vi "Actor Core.vi"(8 "error in":errorcluster, 11 "TRExperimentsRaw in":refnum<class "TRExperimentsRaw.lvclass">) -> (0 "error out":errorcluster, 3 "Actor out":refnum<class "Actor.lvclass">)   [LabVIEW 2020, in "Forms.lvlib" / "TRExperimentsRaw.lvclass"]
doc: "The user interface for this panel.\n\n----\nPlease see the following web address for additional documentation and tutorial information:\nhttp://www.mooregoodideas.com/mgi-panel-manager/\n\nAuthor: Derek Trepanier\n\nCopyright (c) 2018, Moore Good Ideas, Inc.\n\nAll rights reserved.\n\nRedistribution and use in source and binary forms, with or without modification, are permitted provided that the following conditions are met:\n\n * Redistributions of source code must retain the above copyright notice, this list of conditions and the following disclaimer.\n * Redistributions in binary form must reproduce the above copyright notice, this list of conditions and the following disclaimer in the documentation and/or other materials provided with the distribution.\n * Neither the name of Moore Good Ideas, Inc. nor the names of its contributors may be used to endorse or promote products derived from this software without specific prior written permission.\n\nTHIS SOFTWARE IS PROVIDED BY THE COPYRIGHT HOLDERS AND CONTRIBUTORS \"AS IS\" AND ANY EXPRESS OR IMPLIED WARRANTIES, INCLUDING, BUT NOT LIMITED TO, THE IMPLIED WARRANTIES OF MERCHANTABILITY AND FITNESS FOR A PARTICULAR PURPOSE ARE DISCLAIMED. IN NO EVENT SHALL THE COPYRIGHT OWNER OR CONTRIBUTORS BE LIABLE FOR ANY DIRECT, INDIRECT, INCIDENTAL, SPECIAL, EXEMPLARY, OR CONSEQUENTIAL DAMAGES (INCLUDING, BUT NOT LIMITED TO, PROCUREMENT OF SUBSTITUTE GOODS OR SERVICES; LOSS OF USE, DATA, OR PROFITS; OR BUSINESS INTERRUPTION) HOWEVER CAUSED AND ON ANY THEORY OF LIABILITY, WHETHER IN CONTRACT, STRICT LIABILITY, OR TORT (INCLUDING NEGLIGENCE OR OTHERWISE) ARISING IN ANY WAY OUT OF THE USE OF THIS SOFTWARE, EVEN IF ADVISED OF THE POSSIBILITY OF SUCH DAMAGE."
uses:
  TRExperimentsRaw.lvclass
  C:/Users/User/Desktop/Raman Program/Database OOP/forms AF/Form Controller/Panel Form Controller.lvclass
  <vilib>/ActorFramework/Actor/Actor.lvclass
  Text Field Info.ctl
  FK Ring Field Info.ctl
  FK Ring Info.ctl
  Open Form.lvclass
  C:/Users/User/Desktop/Raman Program/Database OOP/source/Button/Button.lvclass
  Users.lvclass
  Samples.lvclass
  DataSets.lvclass
  Working Range.lvclass
  Panel Form Controller.lvclass/Panel Form Controller.ctl
  Constructor by Info Cluster Text.vi
  Constructor by Info Cluster FK Ring.vi
  Panel Form Controller.lvclass
  Field.lvclass
panel:
  in  "Add Working Range":bool
  in  "Add Sample":bool
  in  "Add Data Set":bool
  in  "Add User":bool
  in  "Working Range":u16(ring) items=["None"=1]
  in  "Description":string
  in  "Sample":u16(ring) items=["None"=1, "P"=2, "BSP"=3, "R"=4, "OC"=5, "undoped"=6, "A"=7, "S"=8]
  in  "Data Set":u16(ring) items=["Chopper Phase"=1, "Solvent GS Raman"=2, "Raman Chirp Test"=3, "STO GS Raman"=4, "Program Test"=5, "Front vs Back Refl"=6, "OC ES Raman"=7, "CC ES Raman"=8, "Interfacial Water Test"=9]
  in  "User":u16(ring) items=["None"=1, "Michael"=2, "Suryansh"=3, "Ilya"=4, "Hanna"=5, "Tanja"=6]
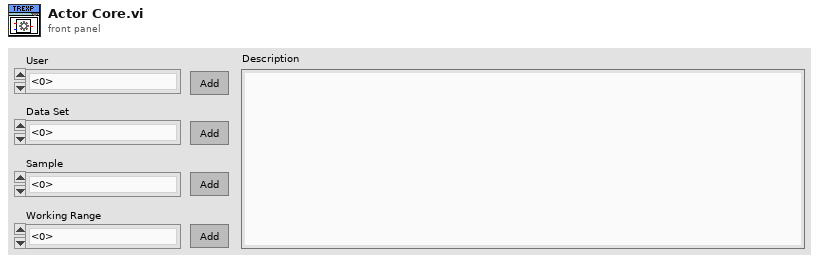
[diagram p1: front panel]
types:
  T1 = typedef "Panel Form Controller.lvlib/Builder Cluster.ctl" = cluster{"Field Map":map{string, refnum<class "Field.lvclass">}, "Button Map":map{string, refnum<class "Button.lvclass">}, "Initialized Field":refnum<class "Field.lvclass">, "VI Ctrl Array":refnum<vi>[]}
  T2 = typedef "Text Field Info.ctl" = cluster{"Ctl Refnum":refnum<vi>, "Table":string, "Column":string}
  T3 = typedef "FK Ring Field Info.ctl" = cluster{"Ctl Refnum":refnum<vi>, "FK Table":string, "FK Column":string, "FK Ring Info":T4}
  T4 = typedef "FK Ring Info.ctl" = cluster{"PK Table":string, "PK Column":string, "PK Display Column":string}
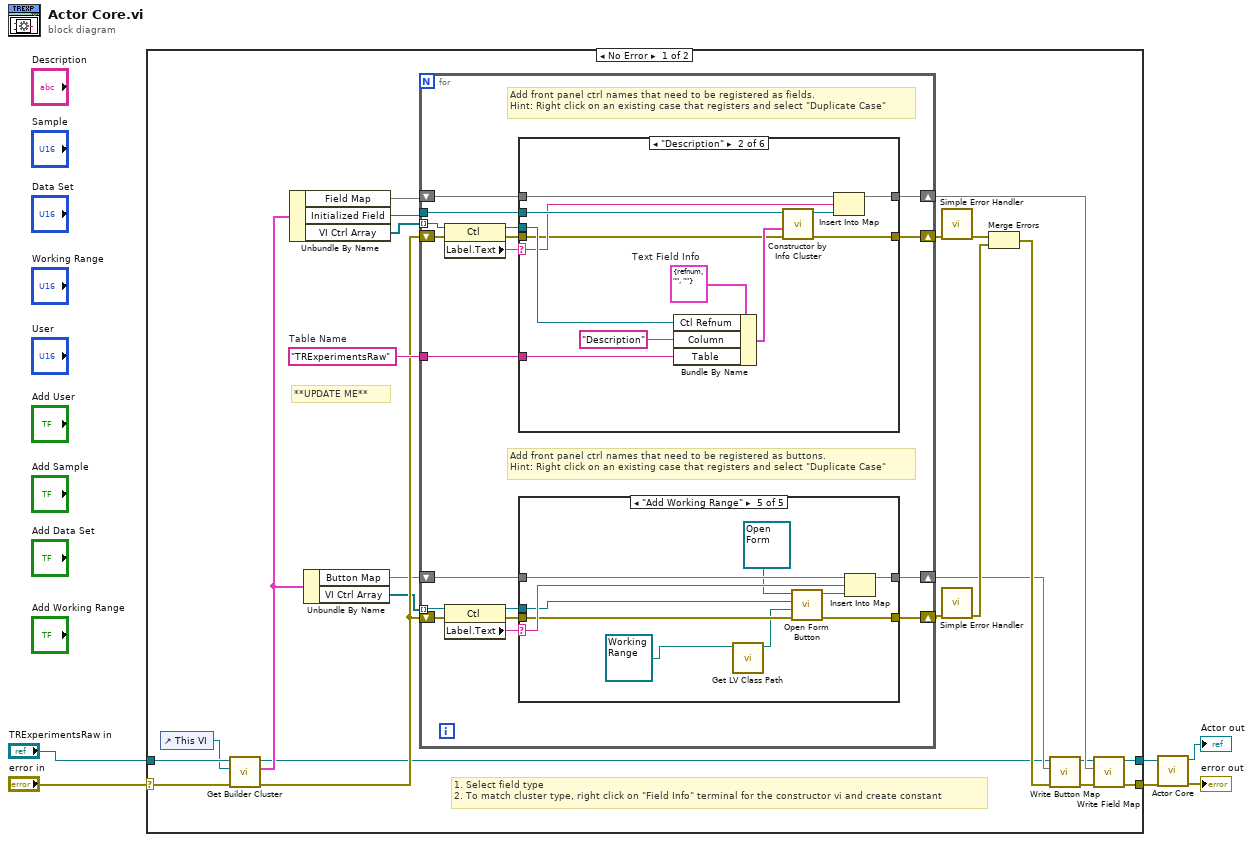
[diagram p0: block diagram]
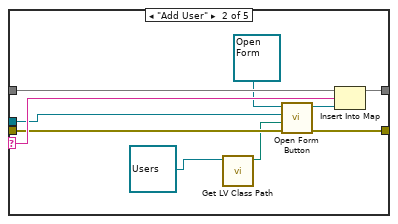
[diagram p3: hidden frame]
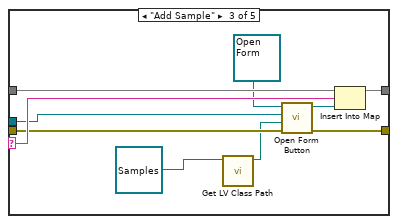
[diagram p4: hidden frame]
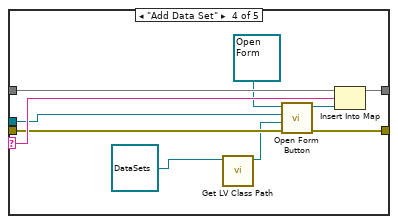
[diagram p5: hidden frame]
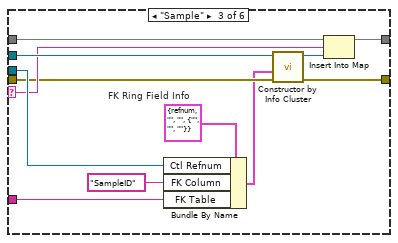
[diagram p7: hidden frame]
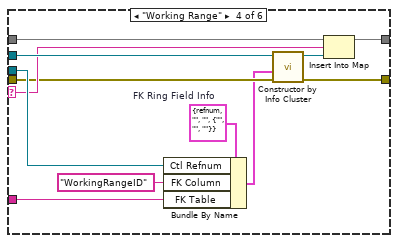
[diagram p8: hidden frame]
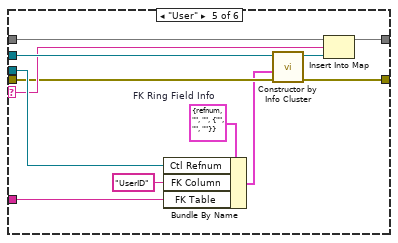
[diagram p9: hidden frame]
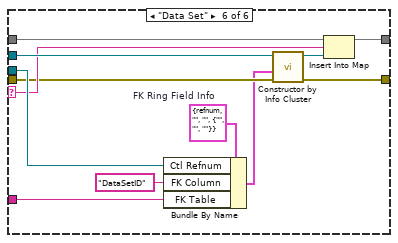
[diagram p10: hidden frame]
diagram:
  n1 = case shown="No Error" "error in" {
    selector: "error in" -> [w10 w153]
    tunnel: "TRExperimentsRaw in" -> [w27 w152]
    tunnel: [w9 w153] -> w4
    tunnel: [w8 w152] -> w3
    frame No Error {
      w29 = "TRExperimentsRaw"  # Table Name
      # "1. Select field type\n2. To match cluster type, right click on \"Field Info\" terminal for the constructor vi and create constant"
      # "**UPDATE ME**"
      n2 = control-ref of="This VI"() -> (w7:refnum<vi>)
      n3 = call "Get Builder Cluster.vi"("error in (no error)"=w10, "VI Refnum"=w7, "Panel Form Controller in"=w27) -> ("error out"=w22:errorcluster, "Builder Cluster"=w20:T1, "Panel Form Controller out"=w11:refnum<class "TRExperimentsRaw.lvclass">)  [unwired: 6 in]
      n4 = Unbundle By Name(w20) -> ("Field Map"=w26:map{string, refnum<class "Field.lvclass">}, "Initialized Field"=w25:refnum<class "Field.lvclass">, "VI Ctrl Array"=w24:refnum<vi>[])
      n5 = Unbundle By Name(w20) -> ("Button Map"=w19:map{string, refnum<class "Button.lvclass">}, "VI Ctrl Array"=w18:refnum<vi>[])
      n6 = for {
        tunnel: w24 -> [w47] mode=indexing
        tunnel: w25 -> [w45]
        tunnel: w29 -> [w44]
        shift-right: [w38] -> w23
        shift-left: w26 -> [w39]
        shift-right: [w43] -> w28
        shift-left: w22 -> [w42]
        shift-right: [w37] -> w21
        shift-left: w22 -> [w36]
        tunnel: w18 -> [w34] mode=indexing
        shift-right: [w31] -> w12
        shift-left: w19 -> [w32]
        # "Add front panel ctrl names that need to be registered as buttons.\nHint: Right click on an existing case that registers and select \"Duplicate Case\""
        # "Add front panel ctrl names that need to be registered as fields.\nHint: Right click on an existing case that registers and select \"Duplicate Case\""
        n7 = property class="Ctl"(reference=w47, error in=w42) -> (reference out=w46:refnum<vi>, error out=w41:errorcluster, "Label.Text"=w40:string)
        n8 = property class="Ctl"(reference=w34, error in=w36) -> (reference out=w33:refnum<vi>, error out=w35:errorcluster, "Label.Text"=w30:string)
        n9 = case shown="\"Description\"" w40 {
          selector: w40 -> [_ w95 w109 w121 w133 w145]
          tunnel: w46 -> [_ w100 w114 w126 w138 w150]
          tunnel: w45 -> [_ w103 w115 w127 w139 w151]
          tunnel: w44 -> [_ w99 w113 w125 w137 w149]
          tunnel: w39 -> [w91 w98 w112 w124 w136 w148]
          tunnel: [w91 w97 w111 w123 w135 w147] -> w38
          tunnel: [w90 w94 w108 w120 w132 w144] -> w43
          tunnel: w41 -> [w90 w93 w107 w119 w131 w143]
          frame "", Default {
          }
          frame "Description" {
            w102 = T2 {"Ctl Refnum"=refnum, "Table"="", "Column"=""}  # Text Field Info
            n10 = Bundle By Name(cluster=w102, "Ctl Refnum"=w100, "Column"="Description", "Table"=w99) -> (w101:T2)
            n11 = call-poly "Constructor by Info Cluster.vi"("error in (no error)"=w93, "Text Field Info"=w101, "Field in"=w103) -> ("error out"=w94:errorcluster, "Field out"=w96:refnum<class "Field.lvclass">)  [unwired: 7 in]
            n12 = Insert Into Map(map in=w98, key=w95, value=w96) -> (map out=w97:map{string, refnum<class "Field.lvclass">})  [unwired: 2 out]
          }
          frame "Sample" {
            w105 = T3 {"Ctl Refnum"=refnum, "FK Table"="", "FK Column"="", "FK Ring Info"={"PK Table"="", "PK Column"="", "PK Display Column"=""}}  # FK Ring Field Info
            n13 = Bundle By Name(cluster=w105, "Ctl Refnum"=w114, "FK Column"="SampleID" ("Column"), "FK Table"=w113) -> (w104:T3)
            n14 = call-poly "Constructor by Info Cluster.vi"("error in (no error)"=w107, "FK Ring Field Info"=w104, "Field in"=w115) -> ("error out"=w108:errorcluster, "Field out"=w110:refnum<class "Field.lvclass">)  [unwired: 7 in]
            n15 = Insert Into Map(map in=w112, key=w109, value=w110) -> (map out=w111:map{string, refnum<class "Field.lvclass">})  [unwired: 2 out]
          }
          frame "Working Range" {
            w117 = T3 {"Ctl Refnum"=refnum, "FK Table"="", "FK Column"="", "FK Ring Info"={"PK Table"="", "PK Column"="", "PK Display Column"=""}}  # FK Ring Field Info
            n16 = Bundle By Name(cluster=w117, "Ctl Refnum"=w126, "FK Column"="WorkingRangeID" ("Column"), "FK Table"=w125) -> (w116:T3)
            n17 = call-poly "Constructor by Info Cluster.vi"("error in (no error)"=w119, "FK Ring Field Info"=w116, "Field in"=w127) -> ("error out"=w120:errorcluster, "Field out"=w122:refnum<class "Field.lvclass">)  [unwired: 7 in]
            n18 = Insert Into Map(map in=w124, key=w121, value=w122) -> (map out=w123:map{string, refnum<class "Field.lvclass">})  [unwired: 2 out]
          }
          frame "User" {
            w129 = T3 {"Ctl Refnum"=refnum, "FK Table"="", "FK Column"="", "FK Ring Info"={"PK Table"="", "PK Column"="", "PK Display Column"=""}}  # FK Ring Field Info
            n19 = Bundle By Name(cluster=w129, "Ctl Refnum"=w138, "FK Column"="UserID" ("Column"), "FK Table"=w137) -> (w128:T3)
            n20 = call-poly "Constructor by Info Cluster.vi"("error in (no error)"=w131, "FK Ring Field Info"=w128, "Field in"=w139) -> ("error out"=w132:errorcluster, "Field out"=w134:refnum<class "Field.lvclass">)  [unwired: 7 in]
            n21 = Insert Into Map(map in=w136, key=w133, value=w134) -> (map out=w135:map{string, refnum<class "Field.lvclass">})  [unwired: 2 out]
          }
          frame "Data Set" {
            w141 = T3 {"Ctl Refnum"=refnum, "FK Table"="", "FK Column"="", "FK Ring Info"={"PK Table"="", "PK Column"="", "PK Display Column"=""}}  # FK Ring Field Info
            n22 = Bundle By Name(cluster=w141, "Ctl Refnum"=w150, "FK Column"="DataSetID" ("Column"), "FK Table"=w149) -> (w140:T3)
            n23 = call-poly "Constructor by Info Cluster.vi"("error in (no error)"=w143, "FK Ring Field Info"=w140, "Field in"=w151) -> ("error out"=w144:errorcluster, "Field out"=w146:refnum<class "Field.lvclass">)  [unwired: 7 in]
            n24 = Insert Into Map(map in=w148, key=w145, value=w146) -> (map out=w147:map{string, refnum<class "Field.lvclass">})  [unwired: 2 out]
          }
        }
        n25 = case shown="\"Add Working Range\"" w30 {
          selector: w30 -> [_ w57 w67 w77 w87]
          tunnel: w33 -> [_ w55 w65 w75 w85]
          tunnel: [w49 w53 w63 w73 w83] -> w37
          tunnel: w35 -> [w49 w54 w64 w74 w84]
          tunnel: w32 -> [w48 w59 w69 w79 w89]
          tunnel: [w48 w58 w68 w78 w88] -> w31
          frame "", Default {
          }
          frame "Add User" {
            n26 = call <vilib>:"Get LV Class Path.vi"("object"=refnum<class "Users.lvclass"> refnum ("Forms.lvlib:Users.lvclass")) -> ("class path"=w51:path)  [unwired: 9 in, 1 out]
            n27 = call "Open Form Button.vi"("error in (no error)"=w54, "Class Path"=w51, "Ctl Refnum"=w55, "Open Form in"=refnum<class "Open Form.lvclass"> refnum) -> ("error out"=w53:errorcluster, "Open Form out"=w56:refnum<class "Open Form.lvclass">)  [unwired: 6 in]
            n28 = Insert Into Map(map in=w59, key=w57, value=w56) -> (map out=w58:map{string, refnum<class "Button.lvclass">})  [unwired: 2 out]
          }
          frame "Add Sample" {
            n29 = call <vilib>:"Get LV Class Path.vi"("object"=refnum<class "Samples.lvclass"> refnum ("Forms.lvlib:Samples.lvclass")) -> ("class path"=w61:path)  [unwired: 9 in, 1 out]
            n30 = call "Open Form Button.vi"("error in (no error)"=w64, "Class Path"=w61, "Ctl Refnum"=w65, "Open Form in"=refnum<class "Open Form.lvclass"> refnum) -> ("error out"=w63:errorcluster, "Open Form out"=w66:refnum<class "Open Form.lvclass">)  [unwired: 6 in]
            n31 = Insert Into Map(map in=w69, key=w67, value=w66) -> (map out=w68:map{string, refnum<class "Button.lvclass">})  [unwired: 2 out]
          }
          frame "Add Data Set" {
            n32 = call <vilib>:"Get LV Class Path.vi"("object"=refnum<class "DataSets.lvclass"> refnum ("Forms.lvlib:DataSets.lvclass")) -> ("class path"=w71:path)  [unwired: 9 in, 1 out]
            n33 = call "Open Form Button.vi"("error in (no error)"=w74, "Class Path"=w71, "Ctl Refnum"=w75, "Open Form in"=refnum<class "Open Form.lvclass"> refnum) -> ("error out"=w73:errorcluster, "Open Form out"=w76:refnum<class "Open Form.lvclass">)  [unwired: 6 in]
            n34 = Insert Into Map(map in=w79, key=w77, value=w76) -> (map out=w78:map{string, refnum<class "Button.lvclass">})  [unwired: 2 out]
          }
          frame "Add Working Range" {
            n35 = call <vilib>:"Get LV Class Path.vi"("object"=refnum<class "Working Range.lvclass"> refnum ("Forms.lvlib:Working Range.lvclass")) -> ("class path"=w81:path)  [unwired: 9 in, 1 out]
            n36 = call "Open Form Button.vi"("error in (no error)"=w84, "Class Path"=w81, "Ctl Refnum"=w85, "Open Form in"=refnum<class "Open Form.lvclass"> refnum) -> ("error out"=w83:errorcluster, "Open Form out"=w86:refnum<class "Open Form.lvclass">)  [unwired: 6 in]
            n37 = Insert Into Map(map in=w89, key=w87, value=w86) -> (map out=w88:map{string, refnum<class "Button.lvclass">})  [unwired: 2 out]
          }
        }
      }
      n38 = call <vilib>:"Simple Error Handler.vi"("error in (no error)"=w28) -> ("error out"=w16:errorcluster)  [unwired: 4 in, 4 out]
      n39 = call <vilib>:"Simple Error Handler.vi"("error in (no error)"=w21) -> ("error out"=w17:errorcluster)  [unwired: 4 in, 4 out]
      n40 = Merge Errors(w16, w17) -> (w15:errorcluster)
      n41 = call "Write Button Map.vi"("error in (no error)"=w15, "Button Map"=w12, "Panel Form Controller in"=w11) -> ("error out"=w14:errorcluster, "Panel Form Controller out"=w13:refnum<class "TRExperimentsRaw.lvclass">)  [unwired: 7 in]
      n42 = call "Write Field Map.vi"("error in (no error)"=w14, "Field Map"=w23, "Panel Form Controller in"=w13) -> ("error out"=w9:errorcluster, "Panel Form Controller out"=w8:refnum<class "TRExperimentsRaw.lvclass">)  [unwired: 7 in]
    }
    frame Error {
    }
  }
  n43 = call-parent "Actor Core.vi"("error in"=w4, "Panel Form Controller in"=w3) -> ("error out"=→"error out":errorcluster, "Actor out"=→"Actor out":refnum<class "Actor.lvclass">)  [unwired: 8 in]
